vi "Set Reference Air Pressure.vi"(8 "error in (no error)":errorcluster, 10 "Reference Air Pressure (0: acutal air pressure)":i32, 11 "Barometer Bricklet in":refnum<class "Barometer Bricklet.lvclass">) -> (0 "error out":errorcluster, 3 "Barometer Bricklet out":refnum<class "Barometer Bricklet.lvclass">)   [LabVIEW 2011, in "Tinkerforge.lvlib" / "Barometer Bricklet.lvclass"]
doc: "This VI sets the reference air pressure in 1/1000 mbar."
uses:
  Barometer Bricklet.lvclass
  Device/Device.lvclass
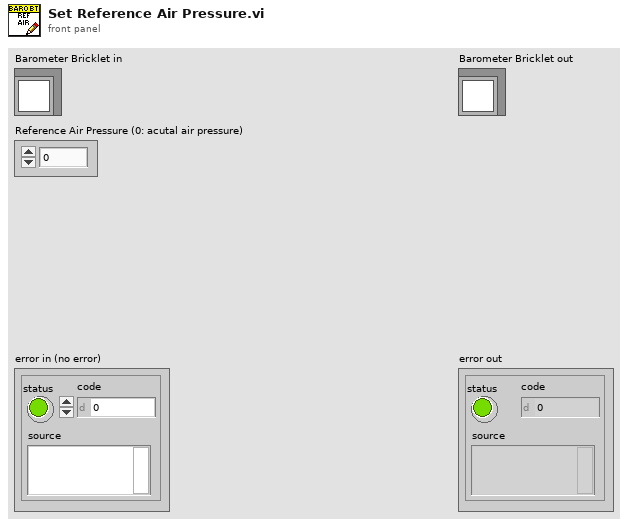
[diagram p1: front panel]
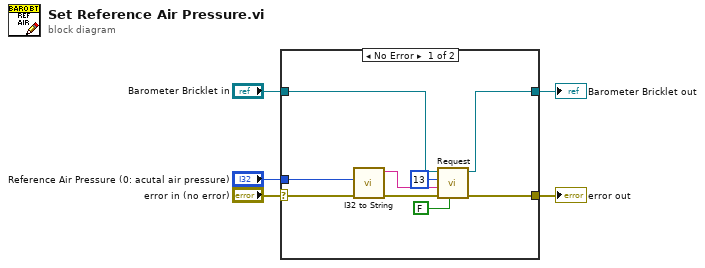
[diagram p0: block diagram]
diagram:
  n1 = case shown="No Error" "error in (no error)" {
    selector: "error in (no error)" -> [w9 w16]
    tunnel: [w10 w16] -> w4
    tunnel: [w13 w15] -> w2
    tunnel: "Barometer Bricklet in" -> [w14 w15]
    tunnel: "Reference Air Pressure (0: acutal air pressure)" -> [w7 _]
    frame No Error {
      n2 = call "I32 to String.vi"("Error In"=w9, "I32"=w7) -> ("Error Out"=w8:errorcluster, "String out"=w6:string)  [unwired: 8 in]
      n3 = call "Request.vi"("Response"=FALSE, "error in (no error)"=w8, "Data"=w6, "Function ID"=u8 13, "Device in"=w14) -> ("error out"=w10:errorcluster, "Device out"=w13:refnum<class "Barometer Bricklet.lvclass">)  [unwired: 2 in, 3 out]
    }
    frame Error {
    }
  }
  "error out" <- w4
  "Barometer Bricklet out" <- w2
